vi "Visual Map.vi"() -> ()   [LabVIEW 2020, in "Pinwheel.lvclass"]
uses:
  Pinwheel.lvclass
panel:
  out "Array 7":u32[][](array[colorbox])=[[9896136, 9896136, 9896136, 9896136, 9896136, 9896136, 9896136, 9896136, 9896136, 9896136, 9896136, 9896136, 9896136, 9896136, 9896136], [9896136, 14643711, 14643711, 14643711, 14643711, 14643711, 14643711, 14643711, 14643711, 14643711, 14643711, 14643711, 14643711, 14643711, 9896136], [9896136, 14643711, 65280, 21760, 39680, 65280, 21760, 39680, 65280, 21760, 39680, 65280, 21760, 14643711, 9896136], [9896136, 14643711, 21760, 39680, 65280, 21760, 39680, 65280, 21760, 39680, 65280, 21760, 39680, 14643711, 9896136], [9896136, 14643711, 39680, 65280, 21760, 39680, 65280, 21760, 39680, 65280, 21760, 39680, 65280, 14643711, 9896136], [9896136, 14643711, 21760, 21760, 39680, 65280, 21760, 39680, 65280, 21760, 39680, 65280, 206, 14643711, 9896136], [9896136, 14643711, 16752816, 39680, 65280, 21760, 39680, 65280, 21760, 39680, 65280, 7829503, 206, 14643711, 9896136], [9896136, 14643711, 16711680, 16752816, 21760, 39680, 65280, 21760, 39680, 65280, 206, 12040191, 7829503, 14643711, 9896136], [9896136, 14643711, 11796481, 16711680, 16752816, 21760, 21760, 39680, 65280, 206, 7829503, 206, 12040191, 14643711, 9896136], [9896136, 14643711, 16752816, 11796481, 16711680, 16752816, 39680, 65280, 7829503, 206, 12040191, 7829503, 206, 14643711, 9896136], [9896136, 14643711, 16711680, 16752816, 11796481, 16711680, 16752816, 16777226, 12040191, 7829503, 206, 12040191, 7829503, 14643711, 9896136], [9896136, 14643711, 11796481, 16711680, 16752816, 11796481, 16711680, 16776607, 16776960, 12040191, 7829503, 206, 12040191, 14643711, 9896136], [9896136, 14643711, 16752816, 11796481, 16711680, 11796481, 16776607, 16776960, 11776768, 11776768, 12040191, 7829503, 206, 14643711, 9896136], [9896136, 14643711, 16711680, 16752816, 11796481, 16776607, 16776960, 11776768, 16776607, 16776960, 11776768, 12040191, 7829503, 14643711, 9896136], [9896136, 14643711, 11796481, 16711680, 16776607, 16776960, 11776768, 16776607, 16776960, 11776768, 16776607, 16776960, 12040191, 14643711, 9896136], [9896136, 14643711, 11796481, 16776607, 16776960, 11776768, 16776607, 16776960, 11776768, 16776607, 16776960, 11776768, 11776768, 14643711, 9896136], [9896136, 14643711, 14643711, 14643711, 14643711, 14643711, 14643711, 14643711, 14643711, 14643711, 14643711, 14643711, 14643711, 14643711, 9896136], [9896136, 9896136, 9896136, 9896136, 9896136, 9896136, 9896136, 9896136, 9896136, 9896136, 9896136, 9896136, 9896136, 9896136, 9896136], [0, 0, 0, 0, 0, 0, 0, 0, 0, 0, 0, 0, 0, 0, 0]]
  out "Array 6":u32[][](array[colorbox])=[[9896136, 9896136, 9896136, 9896136, 9896136, 9896136, 9896136, 9896136, 9896136, 9896136, 9896136, 9896136, 9896136, 9896136, 9896136, 0, 0, 0, 0, 0, 0, 0, 0, 0, 0, 0, 0, 0, 0, 0], [9896136, 14643711, 14643711, 14643711, 14643711, 14643711, 14643711, 14643711, 14643711, 14643711, 14643711, 14643711, 14643711, 14643711, 9896136, 0, 0, 0, 0, 0, 0, 0, 0, 0, 0, 0, 0, 0, 0, 0], [9896136, 14643711, 21760, 39680, 65280, 21760, 39680, 65280, 21760, 39680, 65280, 21760, 39680, 14643711, 9896136, 0, 0, 0, 0, 0, 0, 0, 0, 0, 0, 0, 0, 0, 0, 0], [9896136, 14643711, 39680, 65280, 21760, 39680, 65280, 21760, 39680, 65280, 21760, 39680, 65280, 14643711, 9896136, 0, 0, 0, 0, 0, 0, 0, 0, 0, 0, 0, 0, 0, 0, 0], [9896136, 14643711, 21760, 21760, 39680, 65280, 21760, 39680, 65280, 21760, 39680, 65280, 206, 14643711, 9896136, 0, 0, 0, 0, 0, 0, 0, 0, 0, 0, 0, 0, 0, 0, 0], [9896136, 14643711, 16752816, 39680, 65280, 21760, 39680, 65280, 21760, 39680, 65280, 7829503, 206, 14643711, 9896136, 0, 0, 0, 0, 0, 0, 0, 0, 0, 0, 0, 0, 0, 0, 0], [9896136, 14643711, 16711680, 16752816, 21760, 39680, 65280, 21760, 39680, 65280, 206, 12040191, 7829503, 14643711, 9896136, 0, 0, 0, 0, 0, 0, 0, 0, 0, 0, 0, 0, 0, 0, 0], [9896136, 14643711, 11796481, 16711680, 16752816, 21760, 21760, 39680, 65280, 206, 7829503, 206, 12040191, 14643711, 9896136, 0, 0, 0, 0, 0, 0, 0, 0, 0, 0, 0, 0, 0, 0, 0], [9896136, 14643711, 16752816, 11796481, 16711680, 16752816, 39680, 65280, 7829503, 206, 12040191, 7829503, 206, 14643711, 9896136, 0, 0, 0, 0, 0, 0, 0, 0, 0, 0, 0, 0, 0, 0, 0], [9896136, 14643711, 16711680, 16752816, 11796481, 16711680, 16752816, 16777226, 12040191, 7829503, 206, 12040191, 7829503, 14643711, 9896136, 0, 0, 0, 0, 0, 0, 0, 0, 0, 0, 0, 0, 0, 0, 0], [9896136, 14643711, 11796481, 16711680, 16752816, 11796481, 16711680, 16776607, 16776960, 12040191, 7829503, 206, 12040191, 14643711, 9896136, 0, 0, 0, 0, 0, 0, 0, 0, 0, 0, 0, 0, 0, 0, 0], [9896136, 14643711, 16752816, 11796481, 16711680, 11796481, 16776607, 16776960, 11776768, 11776768, 12040191, 7829503, 206, 14643711, 9896136, 0, 0, 0, 0, 0, 0, 0, 0, 0, 0, 0, 0, 0, 0, 0], [9896136, 14643711, 16711680, 16752816, 11796481, 16776607, 16776960, 11776768, 16776607, 16776960, 11776768, 12040191, 7829503, 14643711, 9896136, 0, 0, 0, 0, 0, 0, 0, 0, 0, 0, 0, 0, 0, 0, 0], [9896136, 14643711, 11796481, 16711680, 16776607, 16776960, 11776768, 16776607, 16776960, 11776768, 16776607, 16776960, 12040191, 14643711, 9896136, 0, 0, 0, 0, 0, 0, 0, 0, 0, 0, 0, 0, 0, 0, 0], [9896136, 14643711, 11796481, 16776607, 16776960, 11776768, 16776607, 16776960, 11776768, 16776607, 16776960, 11776768, 11776768, 14643711, 9896136, 0, 0, 0, 0, 0, 0, 0, 0, 0, 0, 0, 0, 0, 0, 0], [9896136, 14643711, 14643711, 14643711, 14643711, 14643711, 14643711, 14643711, 14643711, 14643711, 14643711, 14643711, 14643711, 14643711, 9896136, 0, 0, 0, 0, 0, 0, 0, 0, 0, 0, 0, 0, 0, 0, 0], [9896136, 9896136, 9896136, 9896136, 9896136, 9896136, 9896136, 9896136, 9896136, 9896136, 9896136, 9896136, 9896136, 9896136, 9896136, 9896136, 9896136, 9896136, 9896136, 9896136, 9896136, 9896136, 9896136, 9896136, 9896136, 9896136, 9896136, 9896136, 9896136, 9896136], [0, 0, 0, 0, 0, 0, 0, 0, 0, 0, 0, 0, 0, 0, 0, 9896136, 3381759, 3381759, 3381759, 3381759, 3381759, 3381759, 3381759, 3381759, 3381759, 3381759, 3381759, 3381759, 3381759, 9896136], [0, 0, 0, 0, 0, 0, 0, 0, 0, 0, 0, 0, 0, 0, 0, 9896136, 3381759, 1870080, 6618880, 9567230, 1870080, 6618880, 9567230, 1870080, 6618880, 9567230, 1870080, 6618880, 3381759, 9896136], [0, 0, 0, 0, 0, 0, 0, 0, 0, 0, 0, 0, 0, 0, 0, 9896136, 3381759, 6618880, 9567230, 1870080, 6618880, 9567230, 1870080, 6618880, 9567230, 1870080, 6618880, 9567230, 14417925, 9896136], [0, 0, 0, 0, 0, 0, 0, 0, 0, 0, 0, 0, 0, 0, 0, 9896136, 14417925, 9567230, 1870080, 6618880, 9567230, 1870080, 6618880, 9567230, 1870080, 6618880, 9567230, 14417925, 0, 9896136], [0, 0, 0, 0, 0, 0, 0, 0, 0, 0, 0, 0, 0, 0, 0, 9896136, 0, 14417925, 6618880, 9567230, 1870080, 6618880, 9567230, 1870080, 6618880, 9567230, 14417925, 0, 0, 9896136], [0, 0, 0, 0, 0, 0, 0, 0, 0, 0, 0, 0, 0, 0, 0, 9896136, 0, 0, 14417925, 1870080, 6618880, 9567230, 1870080, 6618880, 9567230, 14417925, 0, 0, 0, 9896136], [0, 0, 0, 0, 0, 0, 0, 0, 0, 0, 0, 0, 0, 0, 0, 9896136, 0, 0, 0, 14417925, 9567230, 1870080, 6618880, 9567230, 14417925, 0, 0, 0, 0, 9896136], [0, 0, 0, 0, 0, 0, 0, 0, 0, 0, 0, 0, 0, 0, 0, 9896136, 0, 0, 0, 0, 14417925, 6618880, 9567230, 14417925, 0, 0, 0, 0, 0, 9896136], [0, 0, 0, 0, 0, 0, 0, 0, 0, 0, 0, 0, 0, 0, 0, 9896136, 0, 0, 0, 0, 0, 14417925, 16777226, 0, 0, 0, 0, 0, 0, 9896136], [0, 0, 0, 0, 0, 0, 0, 0, 0, 0, 0, 0, 0, 0, 0, 9896136, 0, 0, 0, 0, 0, 0, 0, 0, 0, 0, 0, 0, 0, 9896136], [0, 0, 0, 0, 0, 0, 0, 0, 0, 0, 0, 0, 0, 0, 0, 9896136, 0, 0, 0, 0, 0, 1870080, 6618880, 9567230, 0, 0, 0, 0, 0, 9896136], [0, 0, 0, 0, 0, 0, 0, 0, 0, 0, 0, 0, 0, 0, 0, 9896136, 0, 0, 0, 0, 0, 0, 0, 0, 0, 0, 0, 0, 0, 9896136], [0, 0, 0, 0, 0, 0, 0, 0, 0, 0, 0, 0, 0, 0, 0, 9896136, 0, 0, 0, 0, 0, 0, 0, 0, 0, 0, 0, 0, 0, 9896136], [0, 0, 0, 0, 0, 0, 0, 0, 0, 0, 0, 0, 0, 0, 0, 9896136, 0, 0, 0, 0, 0, 0, 0, 0, 0, 0, 0, 0, 0, 9896136], [0, 0, 0, 0, 0, 0, 0, 0, 0, 0, 0, 0, 0, 0, 0, 9896136, 0, 0, 0, 0, 0, 0, 0, 0, 0, 0, 0, 0, 0, 9896136], [0, 0, 0, 0, 0, 0, 0, 0, 0, 0, 0, 0, 0, 0, 0, 9896136, 9896136, 9896136, 9896136, 9896136, 9896136, 9896136, 9896136, 9896136, 9896136, 9896136, 9896136, 9896136, 9896136, 9896136]]
  out "Array 5":u32[][](array[colorbox])=[[9896136, 9896136, 9896136, 9896136, 9896136, 9896136, 9896136, 9896136, 9896136, 9896136, 9896136, 9896136, 9896136, 9896136, 9896136, 0, 0, 0, 0, 0, 0, 0, 0, 0, 0, 0, 0, 0, 0, 0], [9896136, 14643711, 14643711, 14643711, 14643711, 14643711, 14643711, 14643711, 14643711, 14643711, 14643711, 14643711, 14643711, 14643711, 9896136, 0, 0, 0, 0, 0, 0, 0, 0, 0, 0, 0, 0, 0, 0, 0], [9896136, 14643711, 39680, 65280, 21760, 39680, 65280, 21760, 39680, 65280, 21760, 39680, 65280, 14643711, 9896136, 0, 0, 0, 0, 0, 0, 0, 0, 0, 0, 0, 0, 0, 0, 0], [9896136, 14643711, 21760, 21760, 39680, 65280, 21760, 39680, 65280, 21760, 39680, 65280, 206, 14643711, 9896136, 0, 0, 0, 0, 0, 0, 0, 0, 0, 0, 0, 0, 0, 0, 0], [9896136, 14643711, 16752816, 39680, 65280, 21760, 39680, 65280, 21760, 39680, 65280, 7829503, 206, 14643711, 9896136, 0, 0, 0, 0, 0, 0, 0, 0, 0, 0, 0, 0, 0, 0, 0], [9896136, 14643711, 16711680, 16752816, 21760, 39680, 65280, 21760, 39680, 65280, 206, 12040191, 7829503, 14643711, 9896136, 0, 0, 0, 0, 0, 0, 0, 0, 0, 0, 0, 0, 0, 0, 0], [9896136, 14643711, 11796481, 16711680, 16752816, 21760, 21760, 39680, 65280, 206, 7829503, 206, 12040191, 14643711, 9896136, 0, 0, 0, 0, 0, 0, 0, 0, 0, 0, 0, 0, 0, 0, 0], [9896136, 14643711, 16752816, 11796481, 16711680, 16752816, 39680, 65280, 7829503, 206, 12040191, 7829503, 206, 14643711, 9896136, 0, 0, 0, 0, 0, 0, 0, 0, 0, 0, 0, 0, 0, 0, 0], [9896136, 14643711, 16711680, 16752816, 11796481, 16711680, 16752816, 16777226, 12040191, 7829503, 206, 12040191, 7829503, 14643711, 9896136, 0, 0, 0, 0, 0, 0, 0, 0, 0, 0, 0, 0, 0, 0, 0], [9896136, 14643711, 11796481, 16711680, 16752816, 11796481, 16711680, 16776607, 16776960, 12040191, 7829503, 206, 12040191, 14643711, 9896136, 0, 0, 0, 0, 0, 0, 0, 0, 0, 0, 0, 0, 0, 0, 0], [9896136, 14643711, 16752816, 11796481, 16711680, 11796481, 16776607, 16776960, 11776768, 11776768, 12040191, 7829503, 206, 14643711, 9896136, 0, 0, 0, 0, 0, 0, 0, 0, 0, 0, 0, 0, 0, 0, 0], [9896136, 14643711, 16711680, 16752816, 11796481, 16776607, 16776960, 11776768, 16776607, 16776960, 11776768, 12040191, 7829503, 14643711, 9896136, 0, 0, 0, 0, 0, 0, 0, 0, 0, 0, 0, 0, 0, 0, 0], [9896136, 14643711, 11796481, 16711680, 16776607, 16776960, 11776768, 16776607, 16776960, 11776768, 16776607, 16776960, 12040191, 14643711, 9896136, 0, 0, 0, 0, 0, 0, 0, 0, 0, 0, 0, 0, 0, 0, 0], [9896136, 14643711, 11796481, 16776607, 16776960, 11776768, 16776607, 16776960, 11776768, 16776607, 16776960, 11776768, 11776768, 14643711, 9896136, 0, 0, 0, 0, 0, 0, 0, 0, 0, 0, 0, 0, 0, 0, 0], [9896136, 14643711, 14643711, 14643711, 14643711, 14643711, 14643711, 14643711, 14643711, 14643711, 14643711, 14643711, 14643711, 14643711, 9896136, 0, 0, 0, 0, 0, 0, 0, 0, 0, 0, 0, 0, 0, 0, 0], [9896136, 9896136, 9896136, 9896136, 9896136, 9896136, 9896136, 9896136, 9896136, 9896136, 9896136, 9896136, 9896136, 9896136, 9896136, 0, 0, 0, 0, 0, 0, 0, 0, 0, 0, 0, 0, 0, 0, 0], [0, 0, 0, 0, 0, 0, 0, 0, 0, 0, 0, 0, 0, 0, 0, 9896136, 9896136, 9896136, 9896136, 9896136, 9896136, 9896136, 9896136, 9896136, 9896136, 9896136, 9896136, 9896136, 9896136, 9896136], [0, 0, 0, 0, 0, 0, 0, 0, 0, 0, 0, 0, 0, 0, 0, 9896136, 3381759, 3381759, 3381759, 3381759, 3381759, 3381759, 3381759, 3381759, 3381759, 3381759, 3381759, 3381759, 3381759, 14417925], [0, 0, 0, 0, 0, 0, 0, 0, 0, 0, 0, 0, 0, 0, 0, 14417925, 3381759, 6618880, 9567230, 1870080, 6618880, 9567230, 1870080, 6618880, 9567230, 1870080, 6618880, 9567230, 14417925, 0], [0, 0, 0, 0, 0, 0, 0, 0, 0, 0, 0, 0, 0, 0, 0, 0, 14417925, 9567230, 1870080, 6618880, 9567230, 1870080, 6618880, 9567230, 1870080, 6618880, 9567230, 14417925, 0, 0], [0, 0, 0, 0, 0, 0, 0, 0, 0, 0, 0, 0, 0, 0, 0, 0, 0, 14417925, 6618880, 9567230, 1870080, 6618880, 9567230, 1870080, 6618880, 9567230, 14417925, 0, 0, 0], [0, 0, 0, 0, 0, 0, 0, 0, 0, 0, 0, 0, 0, 0, 0, 0, 0, 0, 14417925, 1870080, 6618880, 9567230, 1870080, 6618880, 9567230, 14417925, 0, 0, 0, 0], [0, 0, 0, 0, 0, 0, 0, 0, 0, 0, 0, 0, 0, 0, 0, 0, 0, 0, 0, 14417925, 9567230, 1870080, 6618880, 9567230, 14417925, 0, 0, 0, 0, 0], [0, 0, 0, 0, 0, 0, 0, 0, 0, 0, 0, 0, 0, 0, 0, 0, 0, 0, 0, 0, 14417925, 6618880, 9567230, 14417925, 0, 0, 0, 0, 0, 0], [0, 0, 0, 0, 0, 0, 0, 0, 0, 0, 0, 0, 0, 0, 0, 0, 0, 0, 0, 0, 0, 14417925, 16777226, 0, 0, 0, 0, 0, 0, 0], [0, 0, 0, 0, 0, 0, 0, 0, 0, 0, 0, 0, 0, 0, 0, 0, 0, 0, 0, 0, 0, 0, 0, 0, 0, 0, 0, 0, 0, 0], [0, 0, 0, 0, 0, 0, 0, 0, 0, 0, 0, 0, 0, 0, 0, 0, 0, 0, 0, 0, 0, 1870080, 6618880, 9567230, 0, 0, 0, 0, 0, 0], [0, 0, 0, 0, 0, 0, 0, 0, 0, 0, 0, 0, 0, 0, 0, 0, 0, 0, 0, 0, 0, 0, 0, 0, 0, 0, 0, 0, 0, 0], [0, 0, 0, 0, 0, 0, 0, 0, 0, 0, 0, 0, 0, 0, 0, 0, 0, 0, 0, 0, 0, 0, 0, 0, 0, 0, 0, 0, 0, 0], [0, 0, 0, 0, 0, 0, 0, 0, 0, 0, 0, 0, 0, 0, 0, 0, 0, 0, 0, 0, 0, 0, 0, 0, 0, 0, 0, 0, 0, 0], [0, 0, 0, 0, 0, 0, 0, 0, 0, 0, 0, 0, 0, 0, 0, 0, 0, 0, 0, 0, 0, 0, 0, 0, 0, 0, 0, 0, 0, 0], [0, 0, 0, 0, 0, 0, 0, 0, 0, 0, 0, 0, 0, 0, 0, 0, 0, 0, 0, 0, 0, 0, 0, 0, 0, 0, 0, 0, 0, 0]]
  out "Array 4":u32[][](array[colorbox])=[[9896136, 9896136, 9896136, 9896136, 9896136, 9896136, 9896136, 9896136, 9896136, 9896136, 9896136, 9896136, 9896136, 9896136, 9896136], [9896136, 14643711, 14643711, 14643711, 14643711, 14643711, 14643711, 14643711, 14643711, 14643711, 14643711, 14643711, 14643711, 14643711, 9896136], [9896136, 14643711, 21760, 21760, 39680, 65280, 21760, 39680, 65280, 21760, 39680, 65280, 206, 14643711, 9896136], [9896136, 14643711, 16752816, 39680, 65280, 21760, 39680, 65280, 21760, 39680, 65280, 7829503, 206, 14643711, 9896136], [9896136, 14643711, 16711680, 16752816, 21760, 39680, 65280, 21760, 39680, 65280, 206, 12040191, 7829503, 14643711, 9896136], [9896136, 14643711, 11796481, 16711680, 16752816, 21760, 21760, 39680, 65280, 206, 7829503, 206, 12040191, 14643711, 9896136], [9896136, 14643711, 16752816, 11796481, 16711680, 16752816, 39680, 65280, 7829503, 206, 12040191, 7829503, 206, 14643711, 9896136], [9896136, 14643711, 16711680, 16752816, 11796481, 16711680, 16752816, 16777226, 12040191, 7829503, 206, 12040191, 7829503, 14643711, 9896136], [9896136, 14643711, 11796481, 16711680, 16752816, 11796481, 16711680, 16776607, 16776960, 12040191, 7829503, 206, 12040191, 14643711, 9896136], [9896136, 14643711, 16752816, 11796481, 16711680, 11796481, 16776607, 16776960, 11776768, 11776768, 12040191, 7829503, 206, 14643711, 9896136], [9896136, 14643711, 16711680, 16752816, 11796481, 16776607, 16776960, 11776768, 16776607, 16776960, 11776768, 12040191, 7829503, 14643711, 9896136], [9896136, 14643711, 11796481, 16711680, 16776607, 16776960, 11776768, 16776607, 16776960, 11776768, 16776607, 16776960, 12040191, 14643711, 9896136], [9896136, 14643711, 11796481, 16776607, 16776960, 11776768, 16776607, 16776960, 11776768, 16776607, 16776960, 11776768, 11776768, 14643711, 9896136], [9896136, 14643711, 14643711, 14643711, 14643711, 14643711, 14643711, 14643711, 14643711, 14643711, 14643711, 14643711, 14643711, 14643711, 9896136], [9896136, 9896136, 9896136, 9896136, 9896136, 9896136, 9896136, 9896136, 9896136, 9896136, 9896136, 9896136, 9896136, 9896136, 9896136]]
  out "Array 10":u32[][](array[colorbox])=[[0, 0, 0, 0, 0, 0, 0, 0, 0, 0, 0, 0, 0, 0, 0], [0, 0, 0, 0, 0, 0, 0, 0, 0, 0, 0, 0, 0, 0, 0], [0, 0, 0, 0, 0, 0, 0, 0, 0, 0, 0, 0, 0, 0, 0], [0, 0, 0, 0, 0, 0, 0, 0, 0, 0, 0, 0, 0, 0, 0], [0, 0, 0, 0, 0, 0, 0, 0, 0, 0, 0, 0, 0, 0, 0], [0, 0, 0, 0, 0, 0, 0, 0, 0, 206, 0, 0, 0, 0, 0], [0, 0, 0, 0, 0, 0, 0, 0, 7829503, 206, 0, 0, 0, 0, 0], [0, 0, 0, 0, 0, 0, 0, 16777226, 0, 7829503, 0, 0, 0, 0, 0], [0, 0, 0, 0, 0, 0, 0, 16776607, 0, 0, 0, 0, 0, 0, 0], [0, 0, 0, 0, 0, 0, 0, 0, 11776768, 11776768, 0, 0, 0, 0, 0], [0, 0, 0, 0, 0, 0, 0, 0, 0, 0, 0, 0, 0, 0, 0], [0, 0, 0, 0, 0, 0, 0, 0, 0, 0, 0, 0, 0, 0, 0], [0, 0, 0, 0, 0, 0, 0, 0, 0, 0, 0, 0, 0, 0, 0], [0, 0, 0, 0, 0, 0, 0, 0, 0, 0, 0, 0, 0, 0, 0], [0, 0, 0, 0, 0, 0, 0, 0, 0, 0, 0, 0, 0, 0, 0]]
  out "Array 9":u32[][](array[colorbox])=[[0, 0, 0, 0, 0, 0, 0, 0, 0, 0, 0, 0, 0, 0, 0], [0, 0, 0, 0, 0, 0, 0, 0, 0, 0, 0, 0, 0, 0, 0], [0, 0, 0, 0, 0, 0, 0, 0, 0, 0, 0, 0, 0, 0, 0], [0, 0, 0, 0, 0, 0, 0, 0, 0, 0, 0, 0, 0, 0, 0], [0, 0, 0, 0, 0, 0, 0, 0, 0, 0, 0, 0, 0, 0, 0], [0, 0, 0, 0, 0, 0, 0, 0, 0, 206, 0, 0, 0, 0, 0], [0, 0, 0, 0, 0, 0, 0, 0, 0, 206, 0, 0, 0, 0, 0], [0, 0, 0, 0, 0, 0, 0, 16777226, 12040191, 0, 0, 0, 0, 0, 0], [0, 0, 0, 0, 0, 0, 0, 0, 0, 0, 0, 0, 0, 0, 0], [0, 0, 0, 0, 0, 0, 0, 0, 0, 0, 0, 0, 0, 0, 0], [0, 0, 0, 0, 0, 0, 0, 0, 0, 0, 0, 0, 0, 0, 0], [0, 0, 0, 0, 0, 0, 0, 0, 0, 0, 0, 0, 0, 0, 0], [0, 0, 0, 0, 0, 0, 0, 0, 0, 0, 0, 0, 0, 0, 0], [0, 0, 0, 0, 0, 0, 0, 0, 0, 0, 0, 0, 0, 0, 0], [0, 0, 0, 0, 0, 0, 0, 0, 0, 0, 0, 0, 0, 0, 0]]
  out "Array 8":u32[][](array[colorbox])=[[0, 0, 0, 0, 0, 0, 0, 0, 0, 0, 0, 0, 0, 0, 0], [0, 0, 0, 0, 0, 0, 0, 0, 0, 0, 0, 0, 0, 0, 0], [0, 0, 0, 0, 0, 0, 0, 0, 0, 0, 0, 0, 0, 0, 0], [0, 0, 0, 0, 0, 0, 0, 0, 0, 0, 0, 0, 0, 0, 0], [0, 0, 0, 0, 0, 0, 0, 0, 0, 0, 0, 0, 0, 0, 0], [0, 0, 0, 0, 0, 0, 0, 0, 0, 0, 0, 0, 0, 0, 0], [0, 0, 0, 0, 0, 0, 0, 65280, 0, 0, 0, 0, 0, 0, 0], [0, 0, 0, 0, 0, 0, 0, 16777226, 0, 0, 0, 0, 0, 0, 0], [0, 0, 0, 0, 0, 0, 0, 0, 0, 0, 0, 0, 0, 0, 0], [0, 0, 0, 0, 0, 0, 0, 0, 0, 0, 0, 0, 0, 0, 0], [0, 0, 0, 0, 0, 0, 0, 0, 0, 0, 0, 0, 0, 0, 0], [0, 0, 0, 0, 0, 0, 0, 0, 0, 0, 0, 0, 0, 0, 0], [0, 0, 0, 0, 0, 0, 0, 0, 0, 0, 0, 0, 0, 0, 0], [0, 0, 0, 0, 0, 0, 0, 0, 0, 0, 0, 0, 0, 0, 0], [0, 0, 0, 0, 0, 0, 0, 0, 0, 0, 0, 0, 0, 0, 0]]
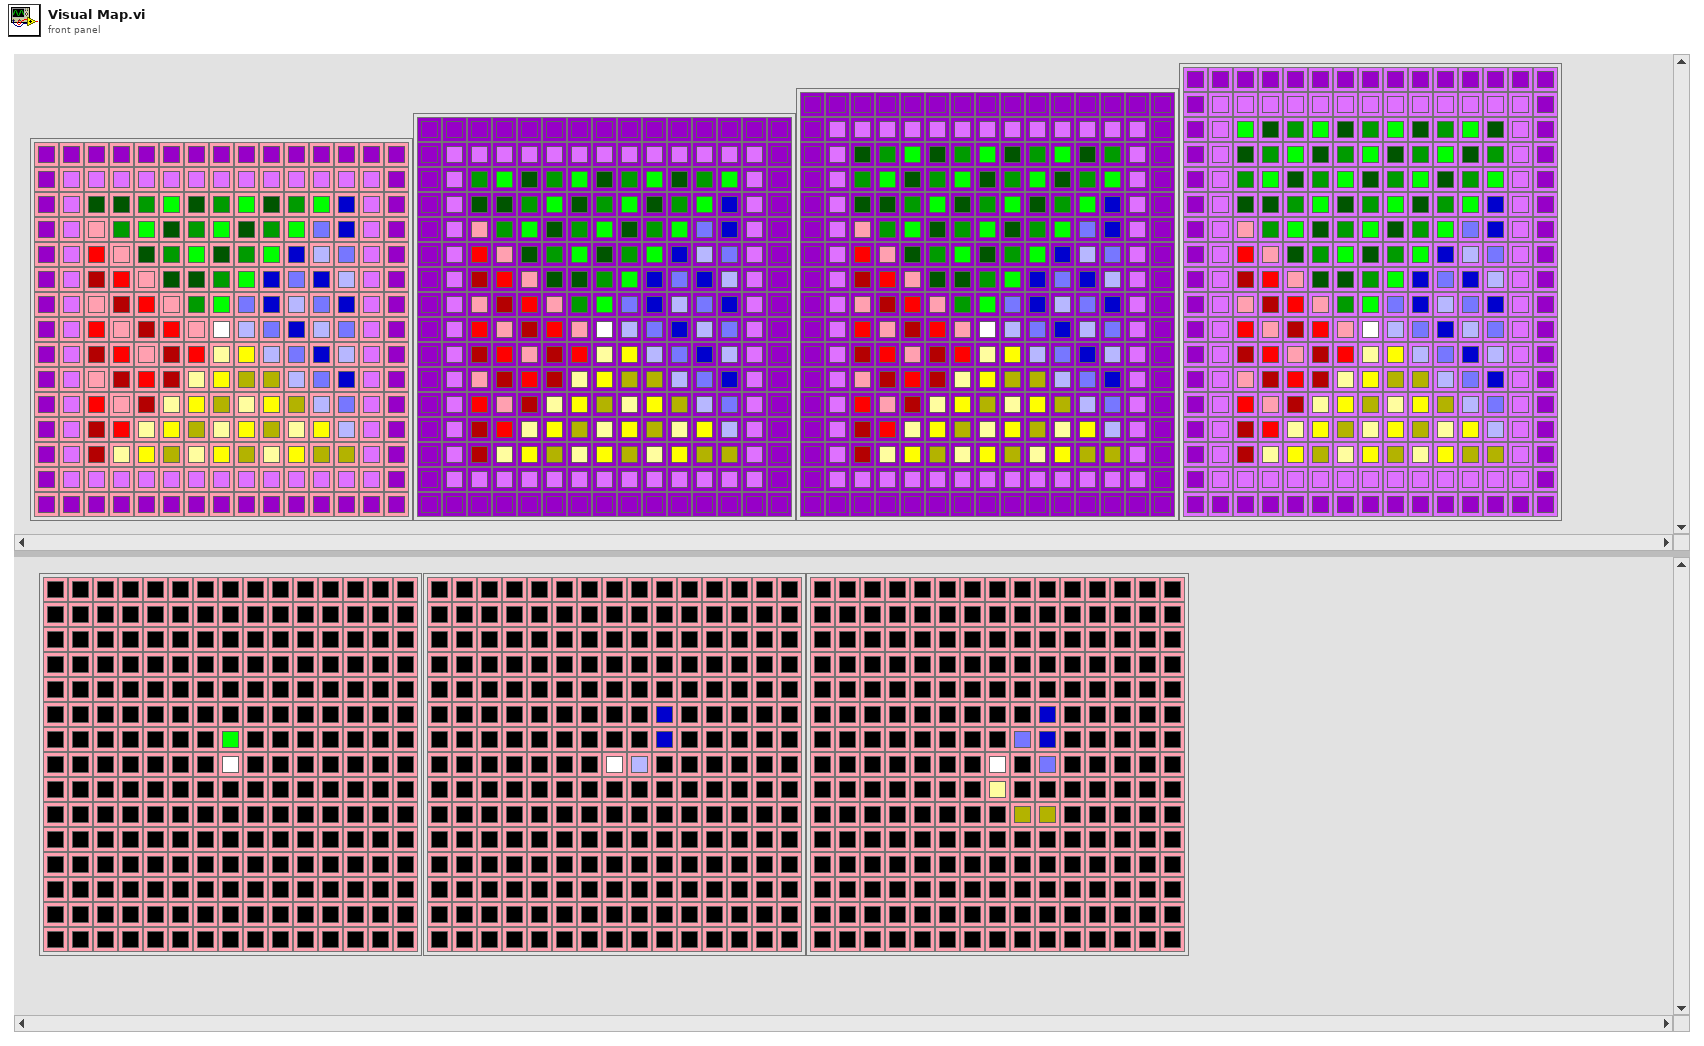
[diagram p1: front panel]
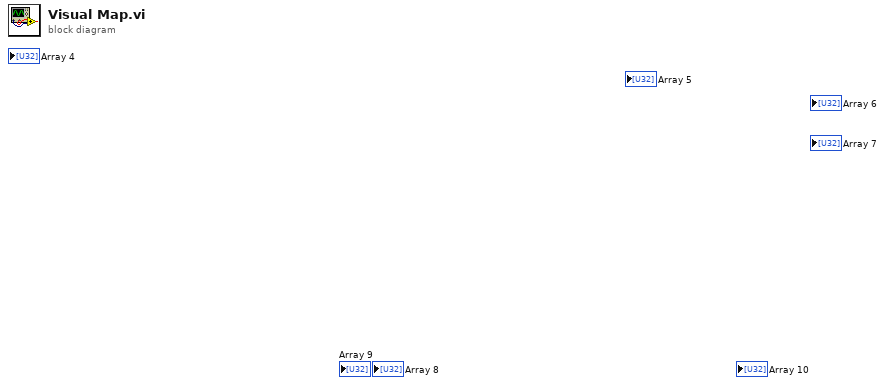
[diagram p0: block diagram]
diagram:
